vi "Enable Phase-Lock Lost Error.vi"(8 "error in (no error)":errorcluster, 10 "Enable Phase-lock Error (T: Enable)":bool=TRUE, 11 "VISA resource name":refnum<visa-resource-name>) -> (0 "error out":errorcluster, 3 "VISA resource name out":refnum<visa-resource-name>)   [LabVIEW 2010, in "AWG.lvlib" / "Agilent 3352X Series.lvlib"]
doc: "Disables or enables the function generator from generating an error if the phase-lock is ever lost by the instrument timebase. Work on both channel.\n\n<b>Note</b>:\n(1) This VI does not check the instrument status. \n(2) The unlock error setting is not stored in non-volatile memory; the setting will be lost when the power is cycled.\n(3) When turn on the phase-lock error, the instrument will generate an error each time the phase locked loop is discovered to be unlocked. A faulty reference signal applied to the 10 MHz IN connector may generate a large number of error messages."
uses:
  Agilent 3352X Series.lvlib
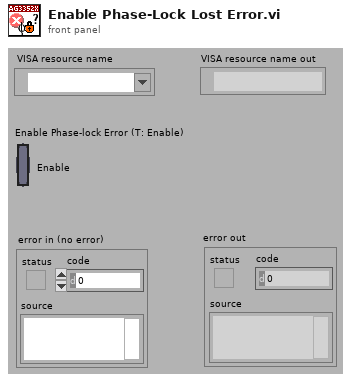
[diagram p1: front panel]
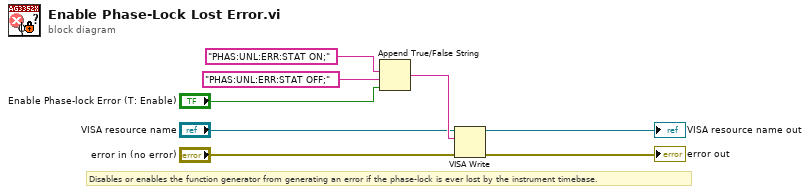
[diagram p0: block diagram]
diagram:
  # "Disables or enables the function generator from generating an error if the phase-lock is ever lost by the instrument timebase."
  n1 = Append True/False String(1:"Enable Phase-lock Error (T: Enable)", 2:"PHAS:UNL:ERR:STAT OFF;", 3:"PHAS:UNL:ERR:STAT ON;") -> (0:w5:string)  [unwired: 1 out]
  n2 = VISA Write(VISA resource name="VISA resource name", write buffer=w5, error in (no error)="error in (no error)") -> (VISA resource name out=→"VISA resource name out":refnum<visa-resource-name>, error out=→"error out":errorcluster)  [unwired: 1 out]
